vi "Motor Controller Command.vi"(8 "error in (no error)":errorcluster, 10 "Command":string, 11 "VISA resource name":refnum<visa-resource-name>) -> (0 "error out":errorcluster, 1 "Timeout on read":bool, 2 "Result":string, 3 "VISA resource name out":refnum<visa-resource-name>)   [LabVIEW 2011]
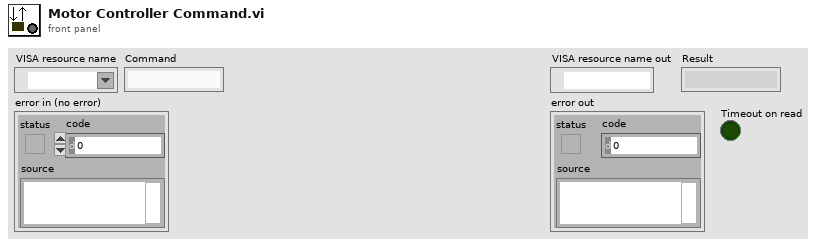
[diagram p1: front panel]
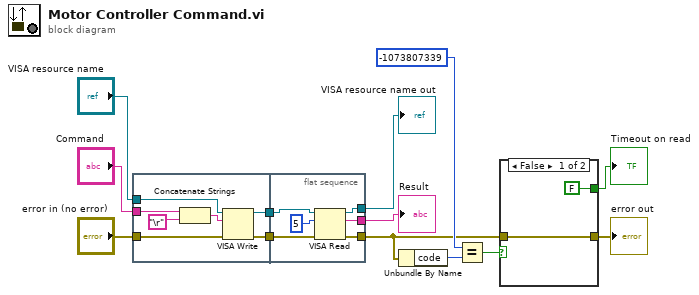
[diagram p0: block diagram]
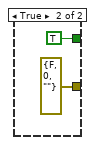
[diagram p2: hidden frame]
diagram:
  n1 = flat-sequence {
    tunnel: [w20] -> w9
    tunnel: [w19] -> w8
    tunnel: "Command" -> [w16]
    tunnel: "VISA resource name" -> [w15]
    tunnel: "error in (no error)" -> [w14]
    tunnel: w9 -> [w26]
    tunnel: [w25] -> w10
    tunnel: w8 -> [w24]
    tunnel: [w23] -> w1
    tunnel: [w21] -> w11
    frame #0 {
      n2 = Concatenate Strings(w16, "\r") -> (w17:string)
      n3 = VISA Write(VISA resource name=w15, write buffer=w17, error in (no error)=w14) -> (VISA resource name out=w20:refnum<visa-resource-name>, error out=w19:errorcluster)  [unwired: 1 out]
    }
    frame #1 {
      n4 = VISA Read(VISA resource name=w26, byte count=u32 5, error in (no error)=w24) -> (VISA resource name out=w25:refnum<visa-resource-name>, read buffer=w21:string, error out=w23:errorcluster)  [unwired: 1 out]
    }
  }
  n5 = Unbundle By Name(w1) -> ("code"=w5:i32)
  n6 = Equal?(x=-1073807339, y=w5) -> (x = y?=w4:bool)
  n7 = case shown="False" w4 {
    tunnel: [FALSE TRUE] -> w3
    tunnel: [w27 errorcluster {"status"=FALSE, "code"=0, "source"=""} ("error out")] -> w2
    tunnel: w1 -> [w27 _]
    frame False {
    }
    frame True {
    }
  }
  "error out" <- w2
  "Timeout on read" <- w3
  "VISA resource name out" <- w10
  "Result" <- w11
